vi "Set Formatter.vi"(8 "error in":errorcluster, 10 "Formatter.lvclass":refnum<class "Formatter.lvclass">, 11 "FileHandler":refnum<class "RotateFileHandler.lvclass">) -> (0 "error out":errorcluster, 3 "FileHandler out":refnum<class "RotateFileHandler.lvclass">)   [LabVIEW 2024, in "RotateFileHandler.lvclass"]
doc: "Sets the Formatter for this handler to fmt.\n\n____\nHAMPEL SOFTWARE ENGINEERING v2.2.2 (2025-01-16 15:41)"
uses:
  RotateFileHandler.lvclass
  <vilib>/Hampel Software Engineering/HSE Logger/Formatter/Formatter.lvclass
  RotateFileHandler.lvclass/RotateFileHandler.ctl
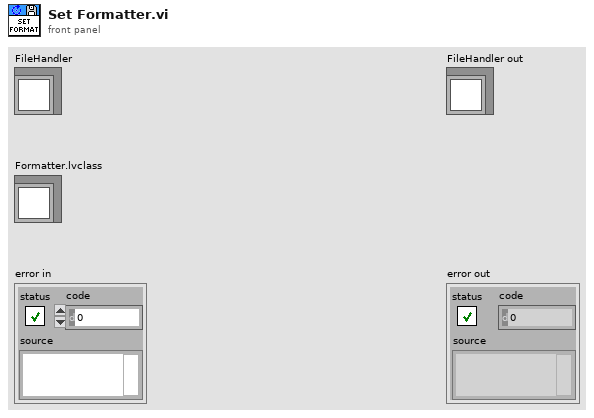
[diagram p1: front panel]
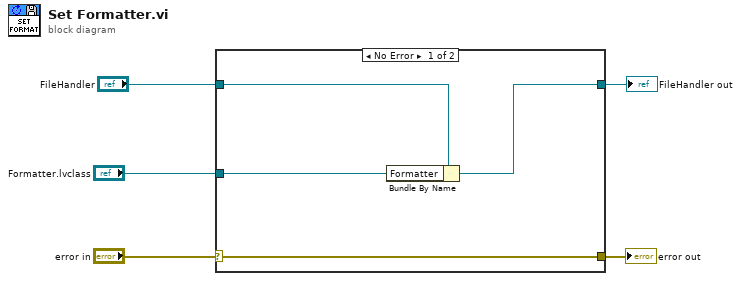
[diagram p0: block diagram]
diagram:
  n1 = case shown="No Error" "error in" {
    selector: "error in" -> [w9 w11]
    tunnel: [w9 w11] -> w4
    tunnel: [w7 w10] -> w1
    tunnel: "FileHandler" -> [w8 w10]
    tunnel: "Formatter.lvclass" -> [w6 _]
    frame No Error {
      n2 = Bundle By Name(cluster=w8, "Formatter"=w6) -> (w7:refnum<class "RotateFileHandler.lvclass">)
    }
    frame Error {
    }
  }
  "error out" <- w4
  "FileHandler out" <- w1
